vi "ME103 Lab1A SP26.vi"() -> ()   [LabVIEW 2025]
uses:
  <vilib>/express/express shared/transition.llb/Dynamic To Waveform Array.vi
  <vilib>/express/express signal manip/GetorSetDDTAttributes/Set DDT Attributes/SetT0.vi
  <vilib>/express/express shared/transition.llb/Waveform Array To Dynamic.vi
  <vilib>/express/express signal manip/GetorSetDDTAttributes/Set DDT Attributes/Set DDT Properties.xnode
panel:
  out "Current Trial":string
  in  "Start Trial":bool
  out "IR Sensor Graph":dynamicdata(graph)
  # "Part 2 - Ping Pong Tower Calibration"
  # "Use this LabVIEW VI to take calibration measurements for the IR sensor in the ping pong tower. \n * IR sensor is located at the top of the ping pong tower\n\nWithin each run, this VI will produce a graph of IR sensor voltages that correspond with the height of the ping pong ball (you and your group will have to measure the distance between the bottom of the sensor to the top of the ping pong ball). Filtering might be required depending on sensor characteristics and noise. \n\nTake at least 10 different ping pong height measurements and graph IR sensor [voltage] vs Ping Pong Distance [cm].  Be sure to compare this against the distance characteristics graph in the IR sensor's datasheet.\n\nNote on Saving Data: Right click on the IR Sensor Graph > Export > Export Data to Excel"
  # "ME 103 Experimentation and Measurements"
  # "Lab 1 Part 2: Ping Pong Tower Calibration"
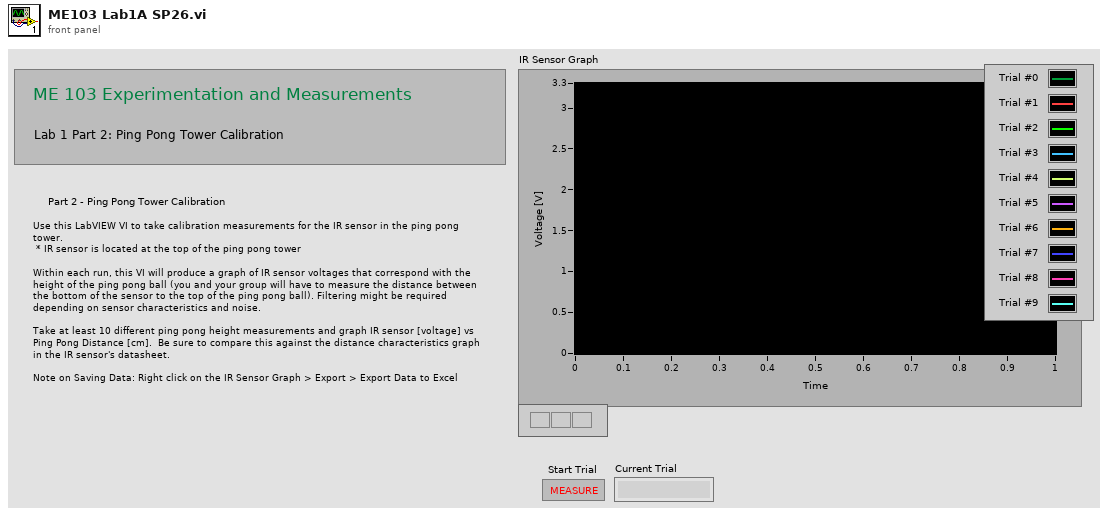
[diagram p1: front panel]
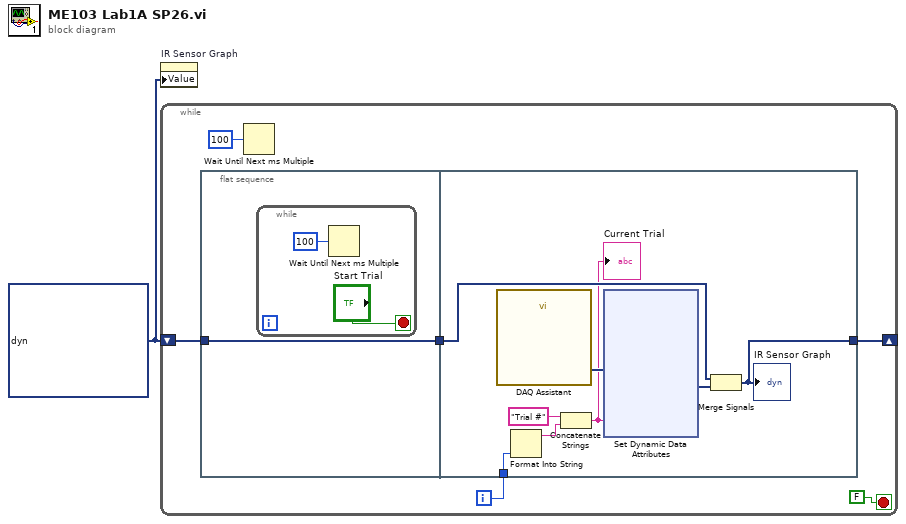
[diagram p0: block diagram]
diagram:
  w1 = dynamicdata [] ("IR Sensor Graph")
  n1 = property on="IR Sensor Graph" class="WFGraph (strict)"("Value"=w1) -> ()  [unwired: 2 in, 2 out]
  n2 = while {
    shift-right: [w7] -> _
    shift-left: w1 -> [w5]
    i -> [w4]
    stop <- FALSE stop-if-true
    n3 = flat-sequence {
      tunnel: [w8] -> w6
      tunnel: w5 -> [w8]
      tunnel: [w17] -> w7
      tunnel: w6 -> [w18]
      tunnel: w4 -> [w16]
      frame #0 {
        n4 = while {
          stop <- "Start Trial" stop-if-true
          n5 = Wait Until Next ms Multiple(millisecond multiple=u32 100) -> ()  [unwired: 1 out]
        }
      }
      frame #1 {
        n6 = call "DAQ Assistant"() -> ("data"=w15:dynamicdata)  [unwired: 17 in, 2 out]
        n7 = Format Into String(w16) -> (resulting string=w13:string)  [unwired: 3 in, 1 out]
        n8 = Concatenate Strings("Trial #" ("string"), w13) -> (w11:string)
        "Current Trial" <- w11
        n9 = xnode "Set Dynamic Data Attributes"("Signals In"=w15, "Signal Name"=w11) -> ("Signals Out"=w14:dynamicdata)  [unwired: 2 in, 1 out]
        n10 = Merge Signals(w18, w14) -> (w17:dynamicdata)
        "IR Sensor Graph" <- w17
      }
    }
    n11 = Wait Until Next ms Multiple(millisecond multiple=u32 100) -> ()  [unwired: 1 out]
  }
